vi "Motors Redefine Origin.vi"(2 "error in":errorcluster, 3 "VISA in":refnum<visa-resource-name>) -> (0 "error out":errorcluster, 1 "VISA out":refnum<visa-resource-name>)   [LabVIEW 2018]
panel:
  out "AP 4":string
  out "AP 3":string
  out "AP 2":string
  out "AP 1":string
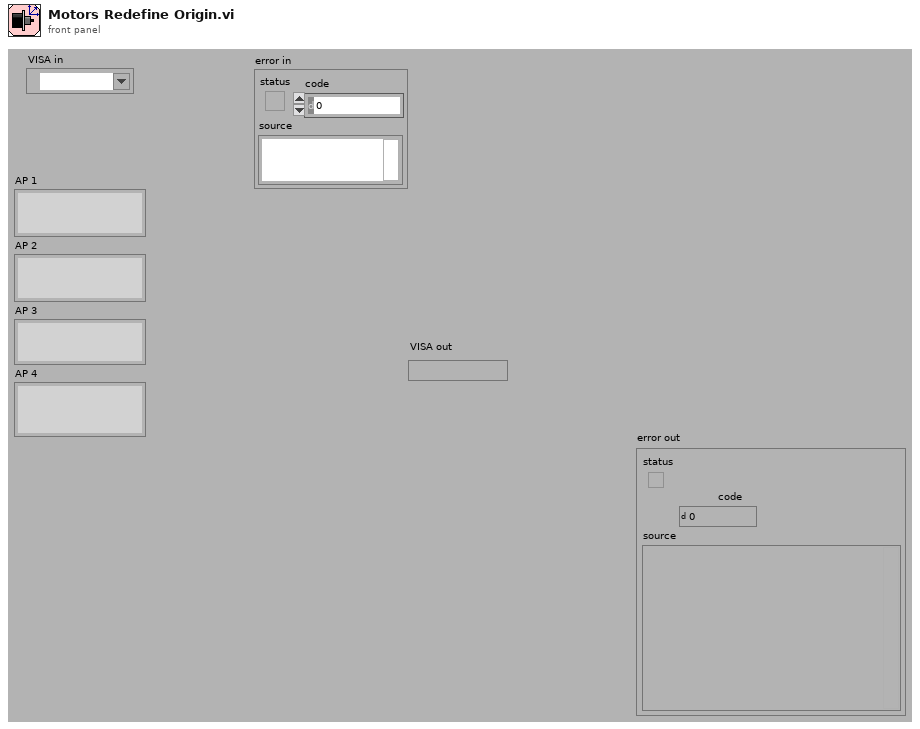
[diagram p1: front panel]
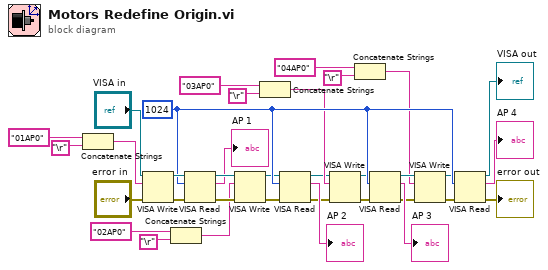
[diagram p0: block diagram]
diagram:
  w27 = u32 1024 ("byte count")
  n1 = Concatenate Strings("01AP0" ("Initial command 1"), "\r") -> (w33:string)
  n2 = VISA Write(VISA resource name="VISA in", write buffer=w33, error in (no error)="error in") -> (VISA resource name out=w31:refnum<visa-resource-name>, error out=w32:errorcluster)  [unwired: 1 out]
  n3 = Concatenate Strings("02AP0" ("Initial command 2"), "\r") -> (w20:string)
  n4 = VISA Read(VISA resource name=w31, byte count=w27, error in (no error)=w32) -> (VISA resource name out=w26:refnum<visa-resource-name>, read buffer=→"AP 1":string, error out=w25:errorcluster)  [unwired: 1 out]
  n5 = VISA Write(VISA resource name=w26, write buffer=w20, error in (no error)=w25) -> (VISA resource name out=w24:refnum<visa-resource-name>, error out=w23:errorcluster)  [unwired: 1 out]
  n6 = Concatenate Strings("03AP0" ("Initial command 3"), "\r") -> (w17:string)
  n7 = VISA Read(VISA resource name=w24, byte count=w27, error in (no error)=w23) -> (VISA resource name out=w15:refnum<visa-resource-name>, read buffer=→"AP 2":string, error out=w16:errorcluster)  [unwired: 1 out]
  n8 = VISA Write(VISA resource name=w15, write buffer=w17, error in (no error)=w16) -> (VISA resource name out=w13:refnum<visa-resource-name>, error out=w14:errorcluster)  [unwired: 1 out]
  n9 = Concatenate Strings("04AP0" ("Initial command 4"), "\r") -> (w7:string)
  n10 = VISA Read(VISA resource name=w13, byte count=w27, error in (no error)=w14) -> (VISA resource name out=w12:refnum<visa-resource-name>, read buffer=→"AP 3":string, error out=w11:errorcluster)  [unwired: 1 out]
  n11 = VISA Write(VISA resource name=w12, write buffer=w7, error in (no error)=w11) -> (VISA resource name out=w9:refnum<visa-resource-name>, error out=w10:errorcluster)  [unwired: 1 out]
  n12 = VISA Read(VISA resource name=w9, byte count=w27, error in (no error)=w10) -> (VISA resource name out=→"VISA out":refnum<visa-resource-name>, read buffer=→"AP 4":string, error out=→"error out":errorcluster)  [unwired: 1 out]
